vi "Do Request.vi"(7 "Processing In":refnum<class "Processing.lvclass">, 11 "ToggleMuteController in":refnum<class "ToggleMuteController.lvclass">) -> (0 "error out":errorcluster, 5 "Processing":refnum<class "Processing.lvclass">)   [LabVIEW 2022 SP3, in "VMR-Deck.lvlib" / "ToggleMuteController.lvclass"]
uses:
  ToggleMuteController.lvclass
  <vilib>/IlluminatedG/IG HTTP Server/HTTP Server/Processing/Processing.lvclass
  ToggleMuteController.lvclass/ToggleMuteController.ctl
  <vilib>/IlluminatedG/IG HTTP Server/HTTP Server/Processing/Processing.lvclass/Processing.ctl
  <vilib>/IlluminatedG/IG VoicemeeterRemote API/VoiceMeeterRemote/Direction.ctl
  <vilib>/IlluminatedG/IG HTTP Utils/HTTP Utils/Request/Request.lvclass
  <vilib>/IlluminatedG/lv-stream/URI/URI.lvclass
  VMR/VMR.lvclass
  <vilib>/IlluminatedG/IG VoicemeeterRemote API/VoiceMeeterRemote/VoiceMeeterRemote.lvlib
  <vilib>/IlluminatedG/IG HTTP Utils/HTTP Utils/Response/Response.lvclass
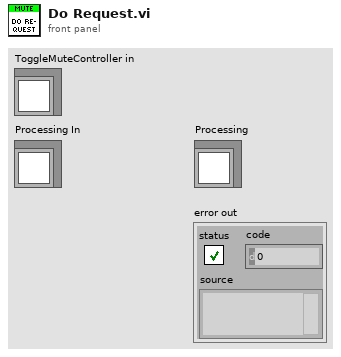
[diagram p1: front panel]
types:
  T1 = typedef "VoiceMeeterRemote.lvlib/Direction.ctl" = enum16{"Input", "Output"}
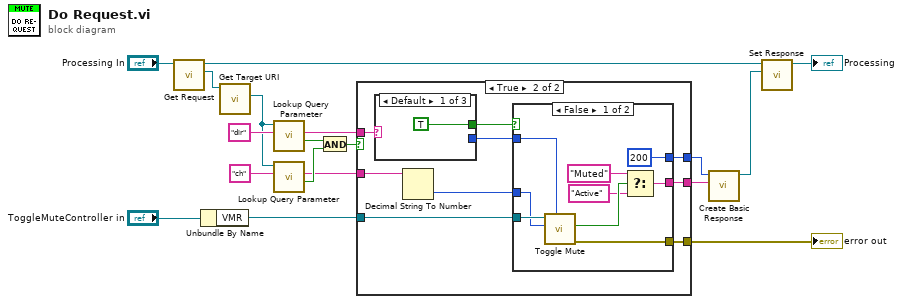
[diagram p0: block diagram]
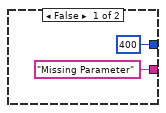
[diagram p2: hidden frame]
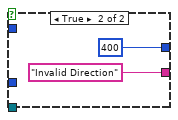
[diagram p3: hidden frame]
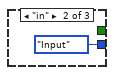
[diagram p4: hidden frame]
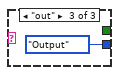
[diagram p5: hidden frame]
diagram:
  n1 = call <vilib>:"Get Request.vi"("Processing in"="Processing In") -> ("Request"=w17:refnum<class "Request.lvclass">, "Processing out"=w3:refnum<class "Processing.lvclass">)  [unwired: 9 in]
  n2 = Unbundle By Name("ToggleMuteController in") -> ("VMR"=w7:refnum<class "VMR.lvclass">)
  n3 = call <vilib>:"Get Target URI.vi"("Request in"=w17) -> ("Target URI"=w14:refnum<class "URI.lvclass">)  [unwired: 8 in, 2 out]
  n4 = call <vilib>:"Lookup Query Parameter.vi"("Name"="dir", "URI in"=w14) -> ("Found"=w13:bool, "Value"=w9:string)  [unwired: 6 in, 2 out]
  n5 = call <vilib>:"Lookup Query Parameter.vi"("Name"="ch", "URI in"=w14) -> ("Found"=w12:bool, "Value"=w10:string)  [unwired: 6 in, 2 out]
  n6 = And(x=w13, y=w12) -> (x .and. y?=w11:bool)
  n7 = case shown="True" w11 {
    tunnel: w10 -> [_ w23]
    tunnel: w9 -> [_ w29]
    tunnel: w7 -> [_ w28]
    tunnel: ["Missing Parameter" ("f") w25] -> w6
    tunnel: [u16 400 w24] -> w5
    tunnel: [_ w21] -> w4
    frame False {
    }
    frame True {
      n8 = case shown="Default" w29 {
        tunnel: [_ Direction."Input" ("Direction") Direction."Output" ("Direction")] -> w27
        tunnel: [TRUE _ _] -> w26
        frame Default {
        }
        frame "in" {
        }
        frame "out" {
        }
      }
      n9 = Decimal String To Number(string=w23) -> (number=w22:i32)  [unwired: 2 in, 1 out]
      n10 = case shown="False" w26 {
        tunnel: w28 -> [w38 _]
        tunnel: w27 -> [w37 _]
        tunnel: [w33 "Invalid Direction" ("f")] -> w25
        tunnel: [u16 200 u16 400] -> w24
        tunnel: w22 -> [w31 _]
        tunnel: [w30 _] -> w21
        frame False {
          n11 = call "Toggle Mute.vi"("Direction"=w37, "Index"=w31, "VMR in"=w38) -> ("error out"=w30:errorcluster, "Muted"=w36:bool)  [unwired: 6 in, 1 out]
          n12 = Select(t="Muted", s=w36, f="Active") -> (s? t:f=w33:string)
        }
        frame True {
        }
      }
    }
  }
  "error out" <- w4
  n13 = call <vilib>:"Create Basic Response.vi"("Payload"=w6, "Status Code"=w5) -> ("Response out"=w1:refnum<class "Response.lvclass">)  [unwired: 8 in, 1 out]
  n14 = call <vilib>:"Set Response.vi"("Response"=w1, "Processing in"=w3) -> ("Processing out"=→"Processing":refnum<class "Processing.lvclass">)  [unwired: 9 in]
